vi "FGV_Voltage Finite Input.vi"() -> ()   [LabVIEW 2017]
doc: "This example demonstrates how to acquire a single buffer of voltage measurements using a DAQmx device.\n\nFor instructions on how to connect your signals to the DAQ device, refer to your device documentation."
uses:
  Controls/FV_Voltage Funite Input.ctl
  <vilib>/DAQmx/read.llb/DAQmx Read (Analog 1D Wfm NChan NSamp).vi
  <vilib>/DAQmx/create/channels.llb/DAQmx Create Channel (AI-Voltage-Basic).vi
  <vilib>/DAQmx/configure/timing.llb/DAQmx Timing (Sample Clock).vi
  <vilib>/DAQmx/configure/task.llb/DAQmx Configure Logging (TDMS).vi
  <vilib>/DAQmx/configure/trigger.llb/DAQmx Start Trigger (Digital Edge).vi
  <vilib>/DAQmx/miscellaneous.llb/DAQmx Fill In Error Info.vi
  <resource>/objmgr/daqmx.rc
panel:
  in  "FV":T1
  in  "Digital Start Trigger Edge":i32(ring)=10280 caption="Edge" items=["Rising"=10280, "Falling"=10171]
  in  "Digital Start Trigger Source":tag="/Dev1/PFI0" caption="Source"
  out "Waveform Graph":waveform(dbl)[](graph)
  in  "TDMS File Path":path
  in  "Number of Samples":i32=100
  in  "Sample Rate":dbl=1000.0
  in  "Sample Clock Source":tag="OnboardClock"
  in  "Terminal Configuration":i32(ring)=-1 items=["default"=-1, "RSE"=10083, "NRSE"=10078, "Differential"=10106, "Pseudodifferential"=12529]
  in  "Max Voltage":dbl=5.0
  in  "Min Voltage":dbl=-5.0
  in  "Physical Channel":tag="Dev1/ai0"
  out "Actual Sample Rate":dbl=1000.0 format="%0.2f"
  in  "Logging Mode":i32(ring)=10231 items=["Off"=10231, "Log and Read"=15842]
  # "Channel Settings"
  # "Acquired Data"
  # "Timing Settings"
  # "Trigger Settings"
  # "Logging Settings"
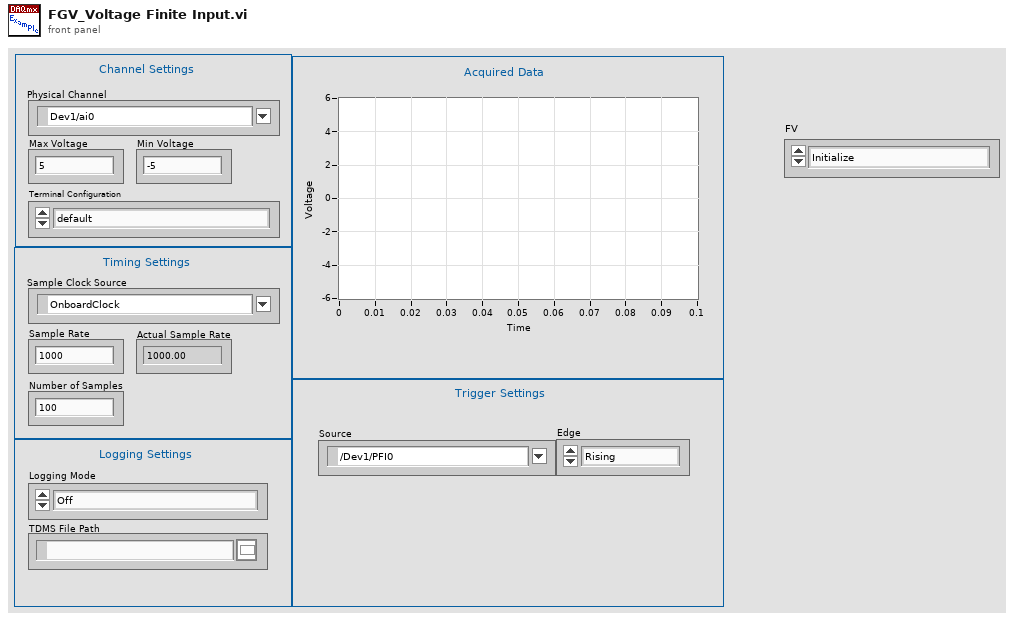
[diagram p1: front panel]
types:
  T1 = typedef "FV_Voltage Funite Input.ctl" = enum16{"Initialize", "Channel Settings", "Timing Settings", "Logging Settings", "Trigger Settings", "Acquire Data", "Task release"}
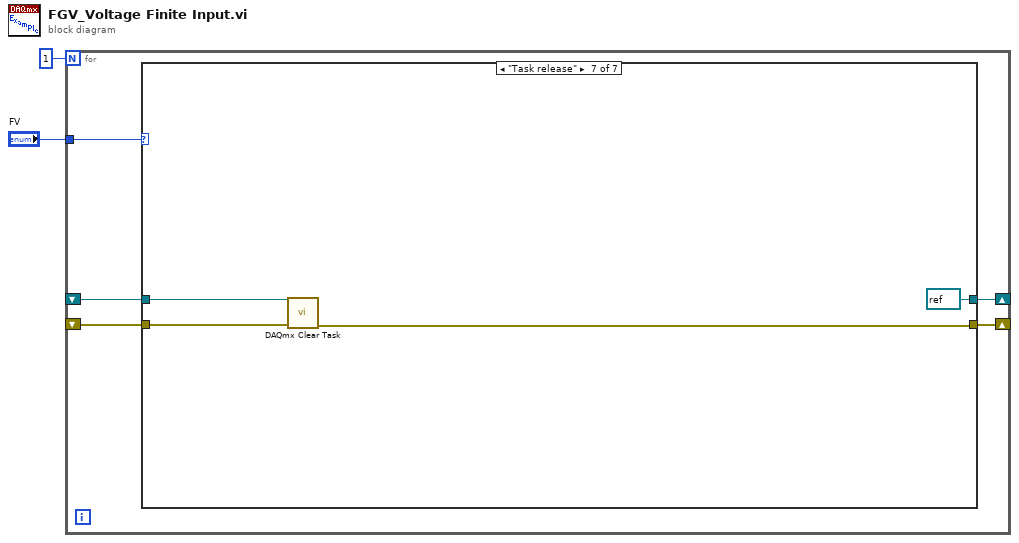
[diagram p0: block diagram]
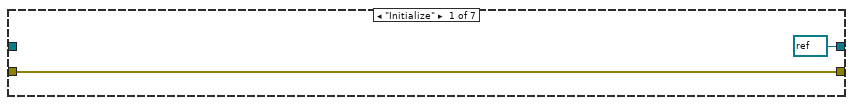
[diagram p2: hidden frame]
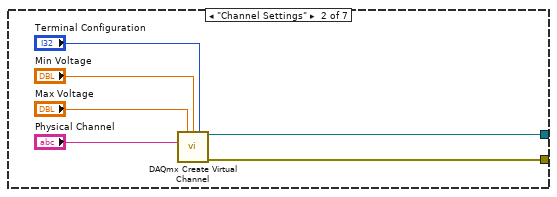
[diagram p3: hidden frame]
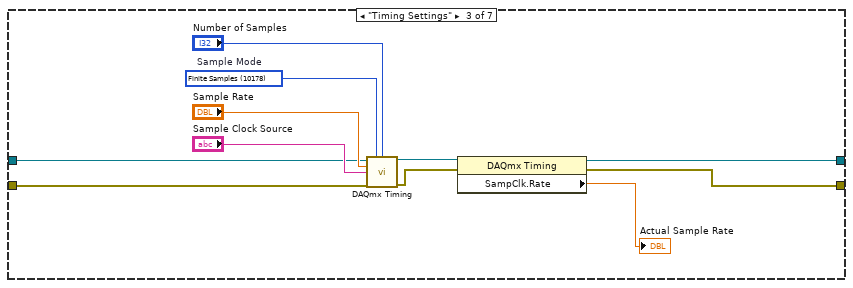
[diagram p4: hidden frame]
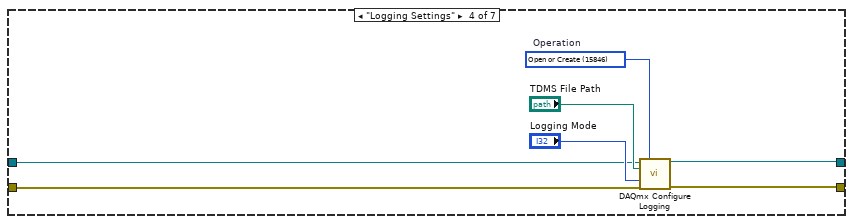
[diagram p5: hidden frame]
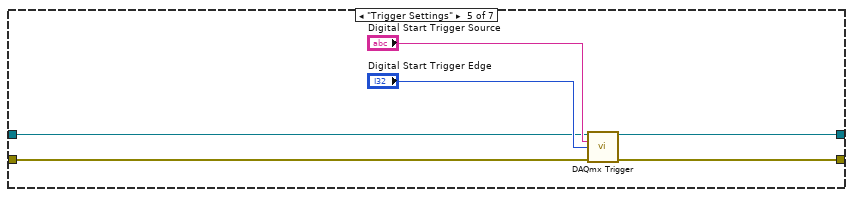
[diagram p6: hidden frame]
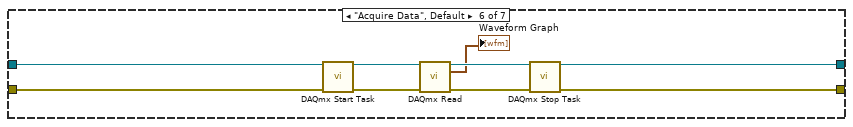
[diagram p7: hidden frame]
diagram:
  n1 = for {
    N: 1 -> [_]
    tunnel: "FV" -> [w7]
    shift-right: [w6] -> _
    shift-left: _ -> [w5]
    shift-right: [w4] -> _
    shift-left: _ -> [w3]
    n2 = case shown="\"Task release\"" w7 {
      tunnel: [refnum<k21> refnum ("task out") w11 w19 w30 w37 w43 refnum<k21> refnum ("task out")] -> w6
      tunnel: w5 -> [_ _ w18 w29 w35 w41 w52]
      tunnel: [w9 w10 w16 w28 w36 w42 w50] -> w4
      tunnel: w3 -> [w9 _ w17 w27 w34 w40 w51]
      frame "Initialize" {
      }
      frame "Channel Settings" {
        n3 = call-poly <vilib>:"DAQmx Create Virtual Channel.vi"("maximum value"="Max Voltage", "minimum value"="Min Voltage", "input terminal configuration"="Terminal Configuration", "physical channels"="Physical Channel") -> ("task out"=w11:refnum<k21>, "error out"=w10:errorcluster)  [unwired: 10 in]
      }
      frame "Timing Settings" {
        w20 = 10178 items=["Finite Samples"=10178, "Continuous Samples"=10123, "Hardware Timed Single Point"=12522]  # Sample Mode
        n4 = call-poly <vilib>:"DAQmx Timing.vi"("task/channels in"=w18, "sample mode"=w20, "samples per channel"="Number of Samples", "rate"="Sample Rate", "source"="Sample Clock Source", "error in"=w17) -> ("task out"=w21:refnum<k21>, "error out"=w22:errorcluster)  [unwired: 8 in]
        n5 = property class="DAQmx Timing"(reference=w21, error in=w22) -> (reference out=w19:refnum<k21>, error out=w16:errorcluster, "SampClk.Rate"=→"Actual Sample Rate":dbl)
      }
      frame "Logging Settings" {
        w31 = 15846 items=["Open"=10437, "Open or Create"=15846, "Create or Replace"=15847, "Create"=15848]  # Operation
        n6 = call-poly <vilib>:"DAQmx Configure Logging.vi"("task/channels in"=w29, "operation"=w31, "file path"="TDMS File Path", "logging mode"="Logging Mode", "error in"=w27) -> ("task out"=w30:refnum<k21>, "error out"=w28:errorcluster)  [unwired: 9 in]
      }
      frame "Trigger Settings" {
        n7 = call-poly <vilib>:"DAQmx Trigger.vi"("task/channels in"=w35, "source"="Digital Start Trigger Source", "edge"="Digital Start Trigger Edge", "error in"=w34) -> ("task out"=w37:refnum<k21>, "error out"=w36:errorcluster)  [unwired: 10 in]
      }
      frame "Acquire Data", Default {
        n8 = call <vilib>:"DAQmx Start Task.vi"("task/channels in"=w41, "error in"=w40) -> ("task out"=w44:refnum<k21>, "error out"=w45:errorcluster)  [unwired: 12 in]
        n9 = call-poly <vilib>:"DAQmx Read.vi"("task/channels in"=w44, "error in"=w45) -> ("task out"=w47:refnum<k21>, "data"=→"Waveform Graph":waveform(dbl)[], "error out"=w48:errorcluster)  [unwired: 11 in]
        n10 = call <vilib>:"DAQmx Stop Task.vi"("task/channels in"=w47, "error in"=w48) -> ("task out"=w43:refnum<k21>, "error out"=w42:errorcluster)  [unwired: 12 in]
      }
      frame "Task release" {
        n11 = call <vilib>:"DAQmx Clear Task.vi"("task in"=w52, "error in"=w51) -> ("error out"=w50:errorcluster)  [unwired: 13 in]
      }
    }
  }
